vi "Configure Standard Offsets.vi"(5 "Standard (1)":i32=1, 6 "Z0  (0.0)":dbl format="%^.2e", 7 "Channel (1)":i32=1, 8 "error in (no error)":errorcluster, 9 "Offset Loss  (0.0)":dbl format="%^.2e", 10 "Offset Delay (0.0)":dbl format="%^.2e", 11 "VISA resource name":refnum<visa-resource-name>) -> (0 "error out":errorcluster, 3 "VISA resource name out":refnum<visa-resource-name>)   [LabVIEW 2011, in "Agilent ENA Series.lvlib"]
doc: "This VI configures calibration kit standard offset."
uses:
  Agilent ENA Series.lvlib
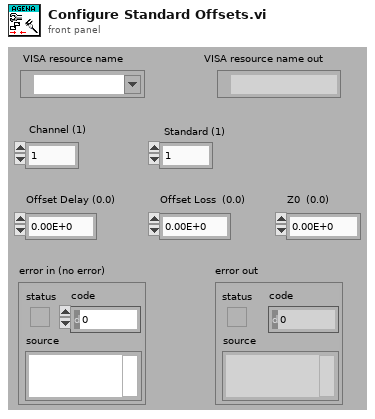
[diagram p1: front panel]
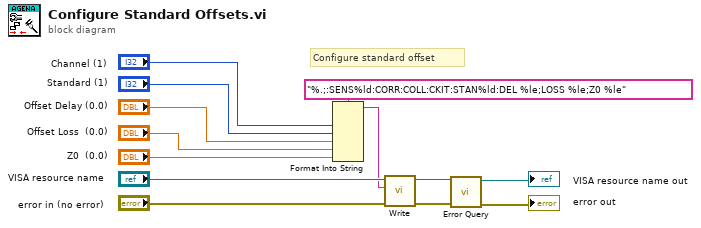
[diagram p0: block diagram]
diagram:
  # "Configure standard offset"
  n1 = Format Into String(format string="%.;:SENS%ld:CORR:COLL:CKIT:STAN%ld:DEL %le;LOSS %le;Z0 %le", "Channel (1)", "Standard (1)", "Offset Delay (0.0)", "Offset Loss  (0.0)", "Z0  (0.0)") -> (resulting string=w10:string)  [unwired: 2 in, 1 out]
  n2 = call "Write.vi"("error in (no error)"="error in (no error)", "String ()"=w10, "VISA resource name"="VISA resource name") -> ("error out"=w3:errorcluster, "VISA resource name out"=w4:refnum<visa-resource-name>)  [unwired: 6 in, 1 out]
  n3 = call "Error Query.vi"("error in (no error)"=w3, "VISA resource name"=w4) -> ("error out"=→"error out":errorcluster, "VISA resource name out"=→"VISA resource name out":refnum<visa-resource-name>)  [unwired: 6 in, 2 out]
